vi "SetAutomaticMode.vi"(0 "Universal Robot.lvclass in":refnum<class "Universal Robot.lvclass">, 5 "error in (no error)":errorcluster) -> (14 "Universal Robot.lvclass out":refnum<class "Universal Robot.lvclass">, 19 "error out":errorcluster)   [LabVIEW 2019, in "Universal Robot.lvclass"]
uses:
  Universal Robot.lvclass
  Universal Robot.lvclass/Universal Robot.ctl
  Client Interfaces/Dashboard Server/Dashboard Server.lvclass
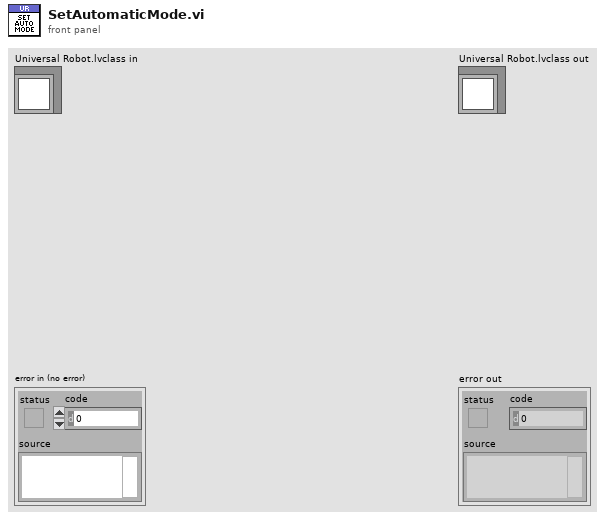
[diagram p1: front panel]
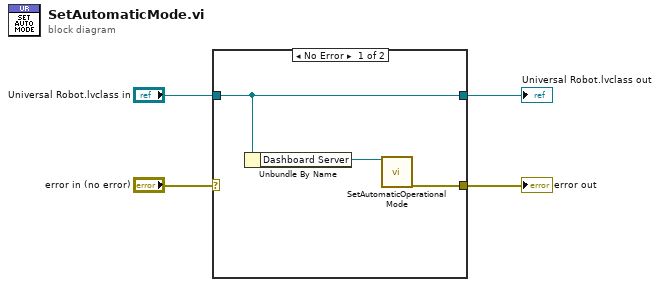
[diagram p0: block diagram]
diagram:
  n1 = case shown="No Error" "error in (no error)" {
    selector: "error in (no error)" -> [_ w9]
    tunnel: [w5 w9] -> w3
    tunnel: "Universal Robot.lvclass in" -> [w7 w8]
    tunnel: [w7 w8] -> w1
    frame No Error {
      n2 = Unbundle By Name(w7) -> ("Dashboard Server"=w6:refnum<class "Dashboard Server.lvclass">)
      n3 = call-dynamic "SetAutomaticOperationalMode.vi"("DashboardServer in"=w6) -> ("error out"=w5:errorcluster)  [unwired: 16 in, 2 out]
    }
    frame Error {
    }
  }
  "error out" <- w3
  "Universal Robot.lvclass out" <- w1
